vi "Cycle_Offset.vi"(2 "Cycle Length":i32, 3 "Step In":i32) -> (0 "Step Out":i32)   [LabVIEW 2014]
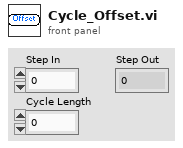
[diagram p1: front panel]
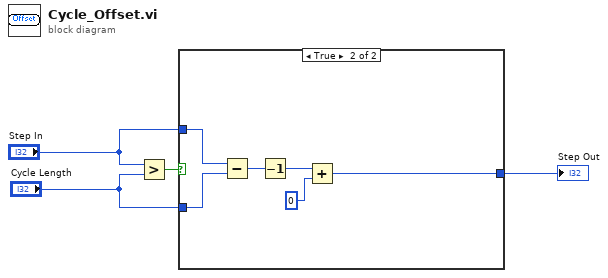
[diagram p0: block diagram]
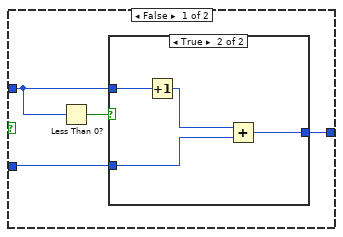
[diagram p2: hidden frame]
diagram:
  n1 = Greater?(x="Step In", y="Cycle Length") -> (0:w3:bool)
  n2 = case shown="True" w3 {
    tunnel: "Cycle Length" -> [w6 w19]
    tunnel: [w5 w15] -> w4
    tunnel: "Step In" -> [w7 w14]
    frame False {
      n3 = Less Than 0?(x=w7) -> (x < 0?=w8:bool)
      n4 = case shown="True" w8 {
        tunnel: [w9 w10] -> w5
        tunnel: w7 -> [w9 w13]
        tunnel: w6 -> [_ w12]
        frame False {
        }
        frame True {
          n5 = Increment(x=w13) -> (x+1=w11:i32)
          n6 = Add(x=w11, y=w12) -> (x+y=w10:i32)
        }
      }
    }
    frame True {
      n7 = Subtract(x=w14, y=w19) -> (x-y=w18:i32)
      n8 = Decrement(x=w18) -> (x-1=w17:i32)
      n9 = Add(x=w17, y=0) -> (x+y=w15:i32)
    }
  }
  "Step Out" <- w4
